vi "cluster2.vi"() -> ()   [LabVIEW 2016]
panel:
  out "output cluster":T1
  out "appended array":dbl[](array[numeric])
  in  "Numeric Control 2":dbl
  in  "String":string
  in  "Boolean":bool
  in  "Numeric Control":dbl
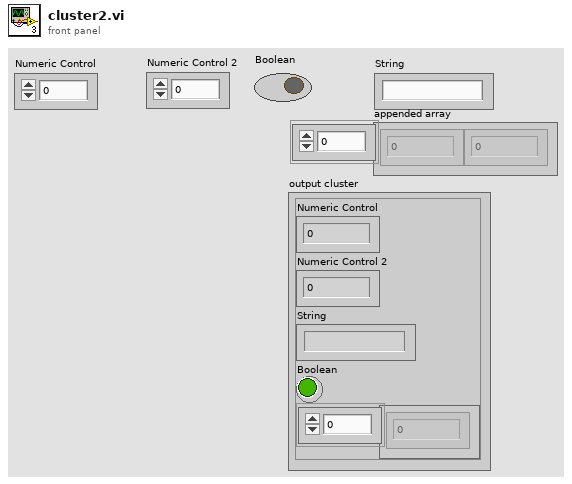
[diagram p1: front panel]
types:
  T1 = cluster{"Numeric Control":dbl, "Numeric Control 2":dbl, "String":string, "Boolean":bool, "Array":dbl[]}
  T2 = cluster{"Numeric Control":dbl, "Numeric Control 2":dbl, "String":string, "Boolean":bool, dbl[]}
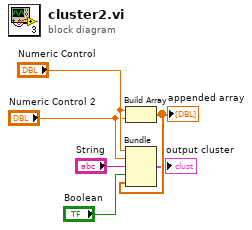
[diagram p0: block diagram]
diagram:
  n1 = Build Array("Numeric Control", "Numeric Control 2") -> (w2:dbl[])
  "appended array" <- w2
  n2 = Bundle("Numeric Control"="Numeric Control", "Numeric Control 2"="Numeric Control 2", "String"="String", "Boolean"="Boolean", w2) -> (→"output cluster":T2)  [unwired: 1 in]
